vi "全局 氨氮.vi"() -> ()   [LabVIEW 2016]
panel:
  in  "氨氮":string[][](array[string])
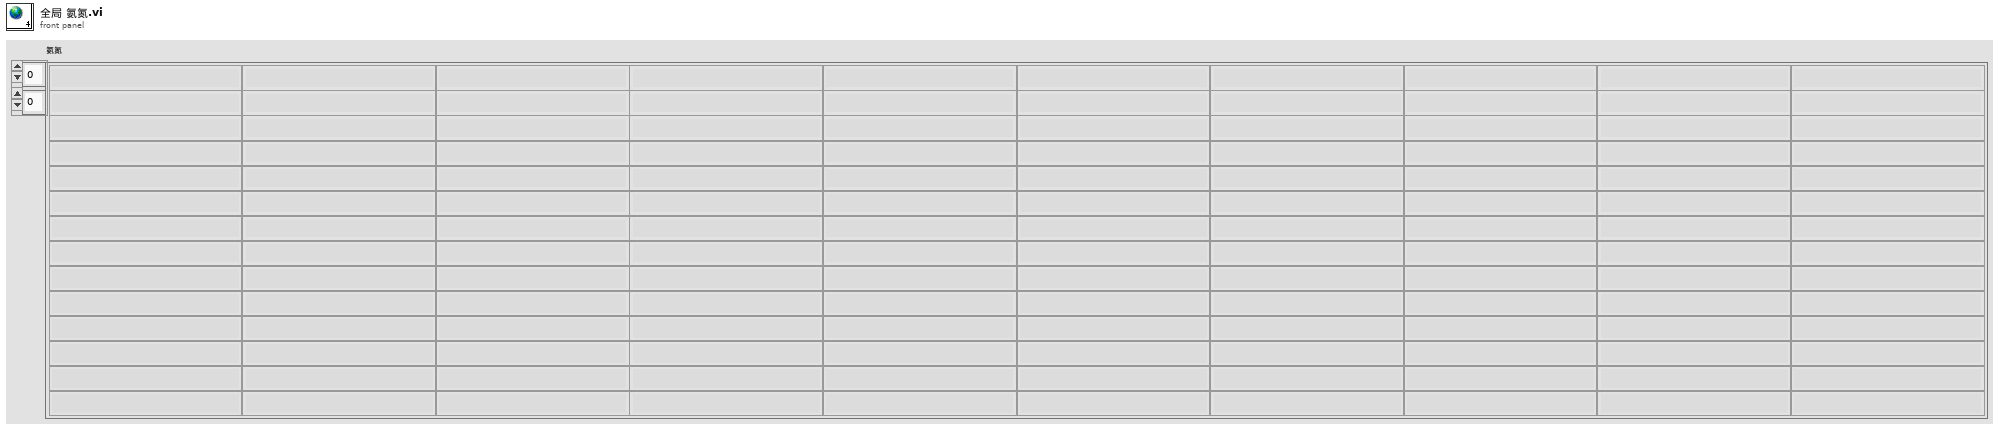
[diagram p1: front panel]
diagram:
